vi "Load Examples.vi"(7 "menu reference":refnum<k9>, 8 "error in (no error)":errorcluster, 11 "Release Name":string) -> (0 "error out":errorcluster)   [LabVIEW 2014]
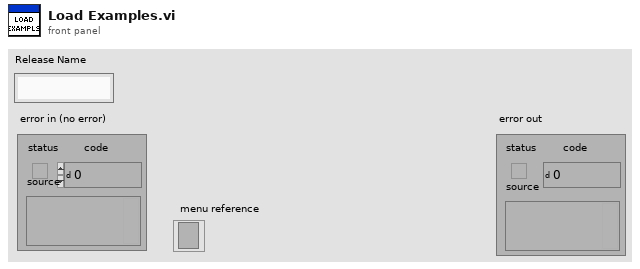
[diagram p1: front panel]
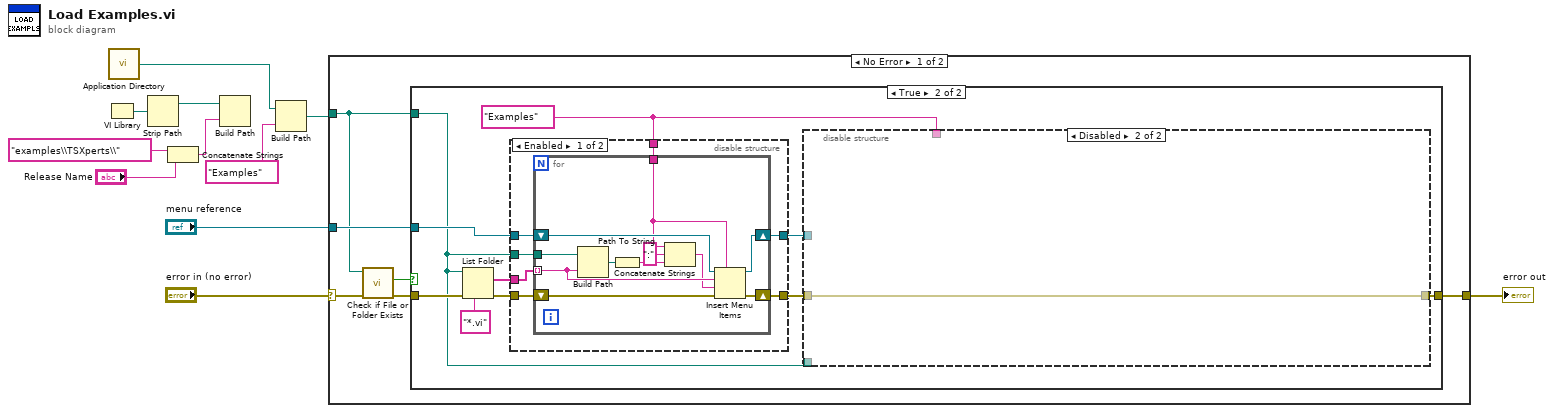
[diagram p0: block diagram]
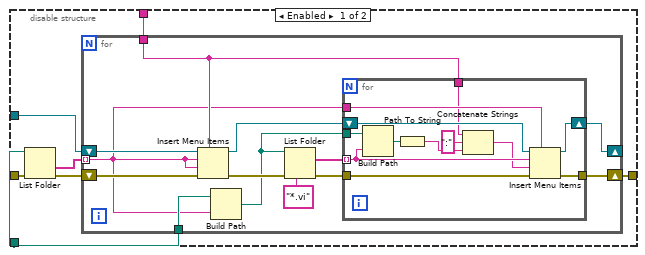
[diagram p3: hidden frame]
diagram:
  n1 = VI Library() -> (path=w8:path)
  n2 = call <vilib>:"Application Directory.vi"() -> ("Application Directory"=w1:path)
  n3 = Strip Path(path=w8) -> (stripped path=w7:path)  [unwired: 1 out]
  n4 = Concatenate Strings("examples\\TSXperts\\" ("name or relative path"), "Release Name") -> (w5:string)
  n5 = Build Path(base path=w7, name or relative path=w5) -> ()  [unwired: 1 out]
  n6 = Build Path(base path=w1, name or relative path="Examples") -> (appended path=w2:path)
  n7 = case shown="No Error" "error in (no error)" {
    selector: "error in (no error)" -> [w15 w82]
    tunnel: [w16 w82] -> w10
    tunnel: "menu reference" -> [w17 _]
    tunnel: w2 -> [w13 _]
    frame No Error {
      n8 = call <vilib>:"Check if File or Folder Exists.vi"("error in (no error)"=w15, "path"=w13) -> ("error out"=w14:errorcluster, "file or folder exists?"=w12:bool)  [unwired: 7 in, 1 out]
      n9 = case shown="True" w12 {
        tunnel: w14 -> [w18 w28]
        tunnel: w17 -> [_ w23]
        tunnel: [w18 w22] -> w16
        tunnel: w13 -> [_ w20]
        frame False {
        }
        frame True {
          w25 = "Examples" ("menu tag")
          n10 = List Folder(path=w20, pattern="*.vi", error in=w28) -> (filenames=w27:string[], error out=w26:errorcluster)  [unwired: 1 in, 2 out]
          n11 = disable-structure shown="Enabled" {
            disable-tunnel: w27 -> [w68 _]
            disable-tunnel: w26 -> [w67 w80]
            disable-tunnel: w25 -> [w66 _]
            disable-tunnel: [w65 w81] -> w24
            disable-tunnel: w23 -> [w64 w81]
            disable-tunnel: [w63 w80] -> w21
            disable-tunnel: w20 -> [w62 _]
            frame Enabled {
              n12 = for {
                tunnel: w68 -> [w74] mode=indexing
                shift-right: [w79] -> w63
                shift-left: w67 -> [w78]
                tunnel: w66 -> [w71]
                shift-right: [w77] -> w65
                shift-left: w64 -> [w76]
                tunnel: w62 -> [w75]
                n13 = Build Path(base path=w75, name or relative path=w74) -> (appended path=w73:path)
                n14 = Path To String(path=w73) -> (string=w72:string)
                n15 = Concatenate Strings(w71, ":" ("string"), w72) -> (w69:string)
                n16 = Insert Menu Items(5:w71, 6:w78, 7:w69, 8:w74, 9:w76) -> (0:w79:errorcluster, 3:w77:refnum<k9>)  [unwired: 1 in, 1 out]
              }
            }
            frame Disabled {
            }
          }
          n17 = disable-structure shown="Disabled" {
            disable-tunnel: w25 -> [w35 _]
            disable-tunnel: w24 -> [w34 _]
            disable-tunnel: [w33 w61] -> w22
            disable-tunnel: w21 -> [w32 w61]
            disable-tunnel: w20 -> [w29 _]
            frame Enabled {
              n18 = List Folder(path=w29, error in=w32) -> (folder names=w30:string[], error out=w31:errorcluster)  [unwired: 2 in, 2 out]
              n19 = for {
                shift-right: [w48] -> w33
                shift-left: w31 -> [w47]
                tunnel: w30 -> [w36] mode=indexing
                tunnel: w35 -> [w37]
                shift-right: [w45] -> _
                shift-left: w34 -> [w46]
                tunnel: w29 -> [w43]
                n20 = Insert Menu Items(5:w37, 6:w47, 7:w36, 8:w36, 9:w46) -> (0:w44:errorcluster, 3:w39:refnum<k9>)  [unwired: 1 in, 1 out]
                n21 = Build Path(base path=w43, name or relative path=w36) -> (appended path=w38:path)
                n22 = List Folder(path=w38, pattern="*.vi", error in=w44) -> (filenames=w40:string[], error out=w41:errorcluster)  [unwired: 1 in, 2 out]
                n23 = for {
                  tunnel: [w60] -> w48
                  tunnel: w41 -> [w58]
                  tunnel: w40 -> [w54] mode=indexing
                  shift-right: [w59] -> w45
                  shift-left: w39 -> [w57]
                  tunnel: w36 -> [w51]
                  tunnel: w38 -> [w55]
                  tunnel: w37 -> [w50]
                  n24 = Build Path(base path=w55, name or relative path=w54) -> (appended path=w56:path)
                  n25 = Path To String(path=w56) -> (string=w52:string)
                  n26 = Concatenate Strings(w50, ":" ("string"), w52) -> (w49:string)
                  n27 = Insert Menu Items(5:w51, 6:w58, 7:w49, 8:w54, 9:w57) -> (0:w60:errorcluster, 3:w59:refnum<k9>)  [unwired: 1 in, 1 out]
                }
              }
            }
            frame Disabled {
            }
          }
        }
      }
    }
    frame Error {
    }
  }
  "error out" <- w10
